vi "Mat Read Test.vi"() -> ()   [LabVIEW 2015]
uses:
  <userlib>/_matio/level5/Public/Utility/List Variables.llb/List Variables (mat file path).vi
  <userlib>/_matio/level5/Public/Read/Extract Data Element.llb/Extract Data Element (2D Array of Data Element from 2D Array of Cell).vi
  <userlib>/_matio/level5/Public/Read/Extract Data Element.llb/Extract Data Element (1D Array of Double).vi
  <userlib>/_matio/level5.lvlib
panel:
  out "data 3":dbl[](array[numeric])
  out "size(s)":i32[](array[numeric])
  out "data 2":string[][](array[string])
  out "data name":string
  out "data":dbl[](array[numeric])
  out "header text":string
  out "resulting string":string
  out "Variables":T1(array[cluster])
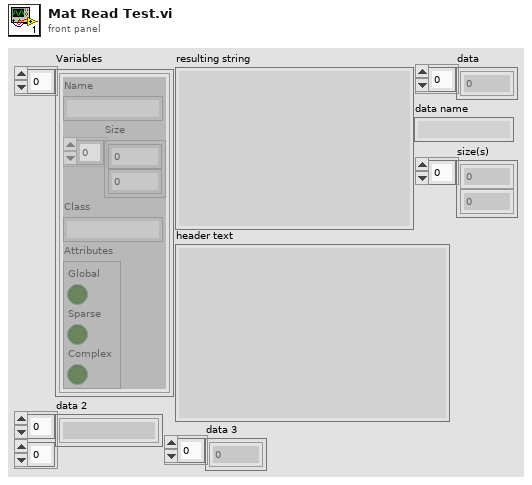
[diagram p1: front panel]
types:
  T1 = cluster{"Name":string, "Size":dbl[], "Class":string, "Attributes":cluster{"Global":bool, "Sparse":bool, "Complex":bool}}[]
  T2 = enum16{"big-endian, network order", "native, host order", "little-endian"}
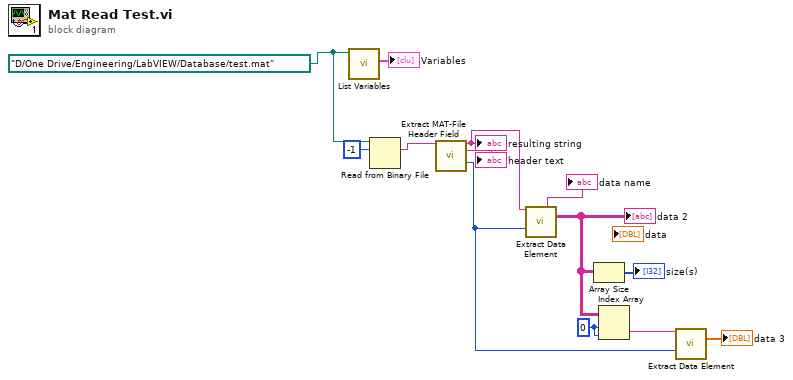
[diagram p0: block diagram]
diagram:
  w4 = 0 ("index (row)")
  w12 = path "D:/One Drive/Engineering/LabVIEW/Database/test.mat" ("file (use dialog)")
  n1 = call-poly <userlib>:"List Variables.vi"("mat string or file path"=w12) -> ("Variables"=→"Variables":T1)  [unwired: 8 in, 2 out]
  n2 = Read from Binary File(10:-1 ("count (1)"), 11:w12) -> (2:w11:string)  [unwired: 4 in, 3 out]
  n3 = call <userlib>:"Extract MAT-File Header Field.vi"("string"=w11) -> ("resulting string"=w8:string, "header text"=→"header text":string, "endian indicator"=w2:T2)  [unwired: 9 in, 3 out]
  "resulting string" <- w8
  n4 = call-poly <userlib>:"Extract Data Element.vi"("string"=w8, "byte order (0:big-endian, network order)"=w2) -> ("data name"=→"data name":string, "data"=w5:string[][])  [unwired: 9 in, 3 out]
  "data 2" <- w5
  n5 = Array Size(array=w5) -> (size(s)=→"size(s)":i32[])
  n6 = Index Array(array=w5, index (row)=w4, index (col)=w4) -> (element=w1:string)
  n7 = call-poly <userlib>:"Extract Data Element.vi"("string"=w1, "byte order (0:big-endian, network order)"=w2) -> ("data"=→"data 3":dbl[])  [unwired: 9 in, 4 out]
